vi "DAQ.Write.vi"(8 "error in (no error)":errorcluster, 10 "Write":T1, 11 "DAQmx in":refnum<class "DAQmx.lvclass">) -> (0 "error out":errorcluster, 3 "DAQmx out":refnum<class "DAQmx.lvclass">)   [LabVIEW 2019]
uses:
  <resource>/objmgr/daqmx.rc
  <vilib>/DAQmx/write.llb/DAQmx Write (Analog 1D Wfm NChan NSamp).vi
  DAQmx.lvclass
  C:/user/patrick/hg/lockin.SMO/lvsrc/DAQ/DAQ.lvclass
  C:/Program Files (x86)/National Instruments/LabVIEW 2016/vi.lib/JKI/JKI SMO/SMO/SMO.lvclass
  DAQ/Typedefs/PrivateEvents--DAQ.Write.ctl
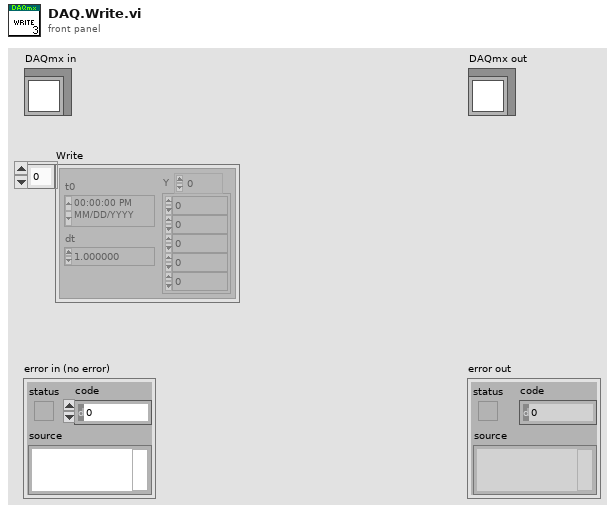
[diagram p1: front panel]
types:
  T1 = typedef "DAQ.lvclass/PrivateEvents--DAQ.Write.ctl" = waveform(dbl)[]
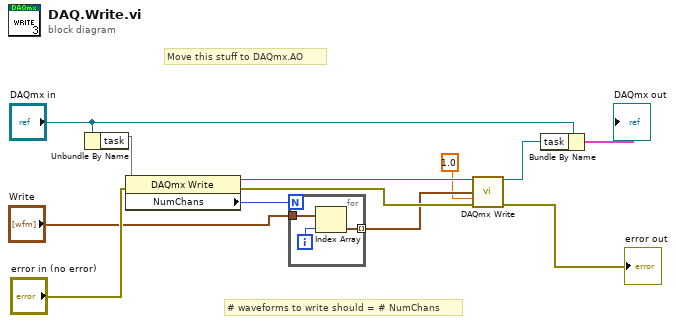
[diagram p0: block diagram]
diagram:
  # "Move this stuff to DAQmx.AO"
  # "# waveforms to write should = # NumChans"
  n1 = Unbundle By Name("DAQmx in") -> ("task"=w1)
  n2 = property class="DAQmx Write"(reference=w1, error in="error in (no error)") -> (reference out=w10:refnum<k21>, error out=w7:errorcluster, "NumChans"=w9:u32)
  n3 = for {
    N: w9 -> [_]
    tunnel: "Write" -> [w15]
    tunnel: [w14] -> w6 mode=indexing
    i -> [w13]
    n4 = Index Array(array=w15, index=w13) -> (element=w14:waveform(dbl))
  }
  n5 = call-poly <vilib>:"DAQmx Write.vi"("task/channels in"=w10, "data"=w6, "timeout"=1.0, "error in"=w7) -> ("task out"=w2:refnum<k21>, "error out"=→"error out":errorcluster)  [unwired: 9 in, 1 out]
  n6 = Bundle By Name(cluster="DAQmx in", "task"=w2) -> (→"DAQmx out":cluster{})
